vi "A_times_x_fxp.vi"(9 "Az_mat in":T2[][](array[typedef]), 10 "x_vec":T1=[0.0, 0.0, 0.0, 0.0, 0.0, 0.0, 0.0, 0.0, 0.0, 0.0, 0.0, 0.0, 0.0, 0.0, 0.0, 0.0, 0.0, 0.0, 0.0, 0.0, 0.0, 0.0, 0.0, 0.0, 0.0]) -> (2 "A*x":T1, 3 "Az_vec out":T2[](array[typedef]))   [LabVIEW 2017]
uses:
  fpga_VIs/fpga_subVIs_ssxy/fixed-point-ss/typeDefs/Az_vec_scalar.ctl
  fpga_VIs/fpga_subVIs_ssxy/fixed-point-ss/typeDefs/x_vec_type.ctl
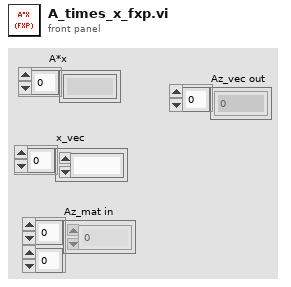
[diagram p1: front panel]
types:
  T1 = typedef "x_vec_type.ctl" = fxp<+/-,32,6>[]
  T2 = typedef "Az_vec_scalar.ctl" = fxp<+/-,32,7>
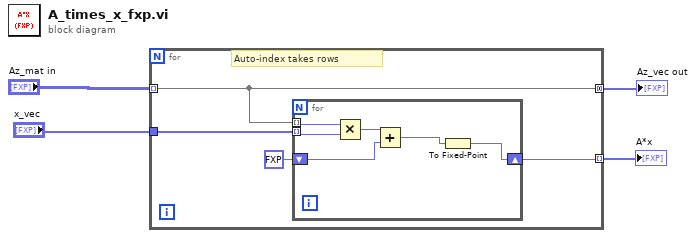
[diagram p0: block diagram]
diagram:
  n1 = for {
    tunnel: "Az_mat in" -> [w8] mode=indexing
    tunnel: [w8] -> w4 mode=concatenating
    tunnel: "x_vec" -> [w7]
    tunnel: [w5] -> w1 mode=indexing
    # "Auto-index takes rows"
    n2 = for {
      tunnel: w8 -> [w14] mode=indexing
      tunnel: w7 -> [w13] mode=indexing
      shift-right: [w9] -> w5
      shift-left: fxp<+,1,1> 0.0 -> [w11]
      n3 = Multiply(x=w14, y=w13) -> (x*y=w12:fxp<+/-,64,13>)
      n4 = Add(x=w12, y=w11) -> (x+y=w10:fxp<+/-,36,13>)
      n5 = To Fixed-Point(number=w10) -> (fixed-point=w9:fxp<+/-,36,13>)  [unwired: 1 in]
    }
  }
  "Az_vec out" <- w4
  "A*x" <- w1
